vi "parseSetForceResponse.vi"(8 "error in (no error)":errorcluster, 10 "DynamicFrameParser":refnum<class "DynamicFrameParser.lvclass">, 11 "DAAILC in":refnum<class "DAAILC.lvclass">) -> (0 "error out":errorcluster, 3 "DAAILC out":refnum<class "DAAILC.lvclass">)   [LabVIEW 2015, in "RTFAILC.lvlib" / "DAAILC.lvclass"]
uses:
  DAAILC.lvclass
  Common_RT_Modbus/DynamicFrameParser/DynamicFrameParser.lvclass
  Common_RT_Modbus/DataTypes/ExceptionCodes.ctl
  FAILC/FAILC.lvclass/FAILC.ctl
  FAILC/FAILC.lvclass
  Common_RT_Modbus/RTModbus.lvlib
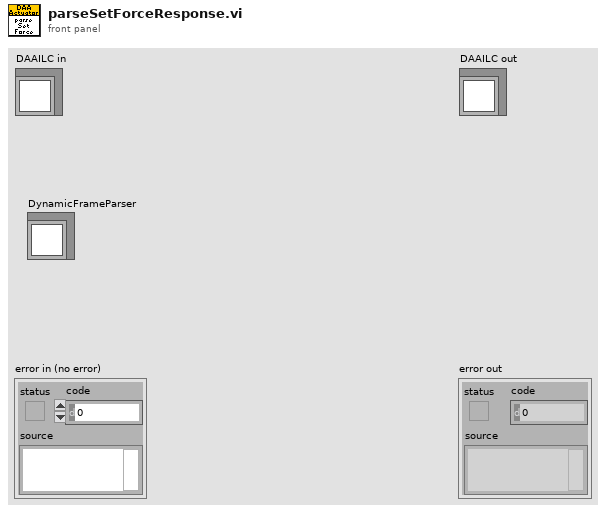
[diagram p1: front panel]
types:
  T1 = typedef "RTModbus.lvlib/ExceptionCodes.ctl" = u16
  T2 = typedef "RTFAILC.lvlib/FAData.ctl" = cluster{"FAConstants":T3, "FACommand":T4, "FATelemetry":T6, "FAResponses":T7}
  T3 = typedef "RTFAILC.lvlib/FAConstants.ctl" = cluster{"ID":i16}
  T4 = typedef "RTFAILC.lvlib/FACommand.ctl" = cluster{"AxialSetPoint":i32, "LateralSetPoint":i32, "PressureServoValveSettings":T5, "BoosterValveSettings":T5}
  T5 = typedef "RTFAILC.lvlib/FAPID.ctl" = cluster{"Kp":sgl, "Ki":sgl, "Kd":sgl, "Kf":sgl}
  T6 = typedef "RTFAILC.lvlib/FATelemetry.ctl" = cluster{"ILCFault":bool, "BroadcastCounter":u8, "AxialLoadCellForce":sgl, "LateralLoadCellForce":sgl, "AxialPressure":T5, "AxialTurbo":T5, "LateralPressure":T5, "LateralTurbo":T5}
  T7 = typedef "RTFAILC.lvlib/FAResponses.ctl" = cluster{"PIDParameters":T1, "ReadPIDParameters":T1, "SetForce":T1, "ForceAndStatus":T1}
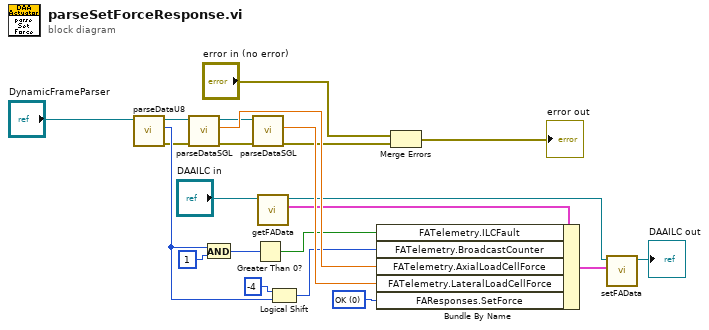
[diagram p0: block diagram]
diagram:
  w1 = T1 0 items=["OK", "IllegalFunction", "IllegalDataAddress", "IllegalDataValue", "SlaveDeviceFailure", "Acknowledge", "SlaveDeviceBusy", "NegativeAcknowledge", "MemoryParityError", "GatewayPathUnavailable", "GatewayTargetDeviceFailedToRespond"] ("FAResponses.ForceAndStatus")
  n1 = call "parseDataU8.vi"("FrameParser in"="DynamicFrameParser") -> ("error out"=w18:errorcluster, "Data"=w20:u8, "FrameParser out"=w16:refnum<class "DynamicFrameParser.lvclass">)  [unwired: 8 in]
  n2 = call "parseDataSGL.vi"("error in (no error)"=w18, "FrameParser in"=w16) -> ("error out"=w12:errorcluster, "Data"=w15:sgl, "FrameParser out"=w13:refnum<class "DynamicFrameParser.lvclass">)  [unwired: 7 in]
  n3 = And(x=w20, y=u8 1) -> (x .and. y?=w21:u8)
  n4 = call "parseDataSGL.vi"("error in (no error)"=w12, "FrameParser in"=w13) -> ("error out"=w11:errorcluster, "Data"=w14:sgl)  [unwired: 7 in, 1 out]
  n5 = Greater Than 0?(x=w21) -> (x > 0?=w3:bool)
  n6 = call "getFAData.vi"("FAILC in"="DAAILC in") -> ("FAData"=w8:T2, "FAILC out"=w6:refnum<class "DAAILC.lvclass">)  [unwired: 9 in]
  n7 = Logical Shift(y=i16 -4, x=w20) -> (x << y=w2:u8)
  n8 = Bundle By Name(cluster=w8, "FATelemetry.ILCFault"=w3, "FATelemetry.BroadcastCounter"=w2, "FATelemetry.AxialLoadCellForce"=w15, "FATelemetry.LateralLoadCellForce"=w14, "FAResponses.SetForce"=w1) -> (w7:T2)
  n9 = Merge Errors("error in (no error)", w11) -> (→"error out":errorcluster)
  n10 = call "setFAData.vi"("FAData"=w7, "FAILC in"=w6) -> ("FAILC out"=→"DAAILC out":refnum<class "DAAILC.lvclass">)  [unwired: 9 in]
